vi "WPs and Obstacles 6.vi"(10 "WP Real Longs":dbl[](array[numeric])=[81.2671, 81.26711, 81.267112, 81.267332, 81.267916, 81.267137, 81.267874, 81.267301, 81.267913, 81.26772] format="%#_8g", 11 "WP Real Lats":dbl[](array[numeric])=[37.1528, 37.15281, 37.152877, 37.152903, 37.152565, 37.152792, 37.152806, 37.152779, 37.152868, 37.152484] format="%#_8g") -> (0 "Obstacle Real Lats and Longs":cluster{"Obs Lats":dbl[], "Obs Longs":dbl[]} {"Obs Longs" format="%#_8g"; "Obs Lats" format="%#_8g"}, 1 "WP Real Lats and Longs":cluster{"WP Lats":dbl[], "WP Longs":dbl[]} {"WP Longs" format="%#_8g"; "WP Lats" format="%#_8g"}, 2 "Sim Matrx":u8[][](array[numeric]), 3 "Real WP Map":T1(graph), 5 "Sim Course":picture)   [LabVIEW 2014]
panel:
  out "Array":dbl[](array[numeric])
  in  "Obstacle Real Longs":dbl[](array[numeric])=[81.2678, 81.267312, 81.267112, 81.267332, 81.267916, 81.267137, 81.267874, 81.267301, 81.267913, 81.26772] format="%#_8g"
  in  "Obstacle Real Lats":dbl[](array[numeric])=[37.1524, 37.152256, 37.152877, 37.152903, 37.152565, 37.152792, 37.152806, 37.152779, 37.152868, 37.152484] format="%#_8g"
  # "Waypoint and Obstacles 6 (Uses Paint and On-Screen WPs)"
  # "Added Global sim painted map"
  # "Inputs:"
  # "Sim Lats and Longs not being used"
  # "20"
  # "12"
  # "Outputs:"
  # "Sim Painted Picture to matrix"
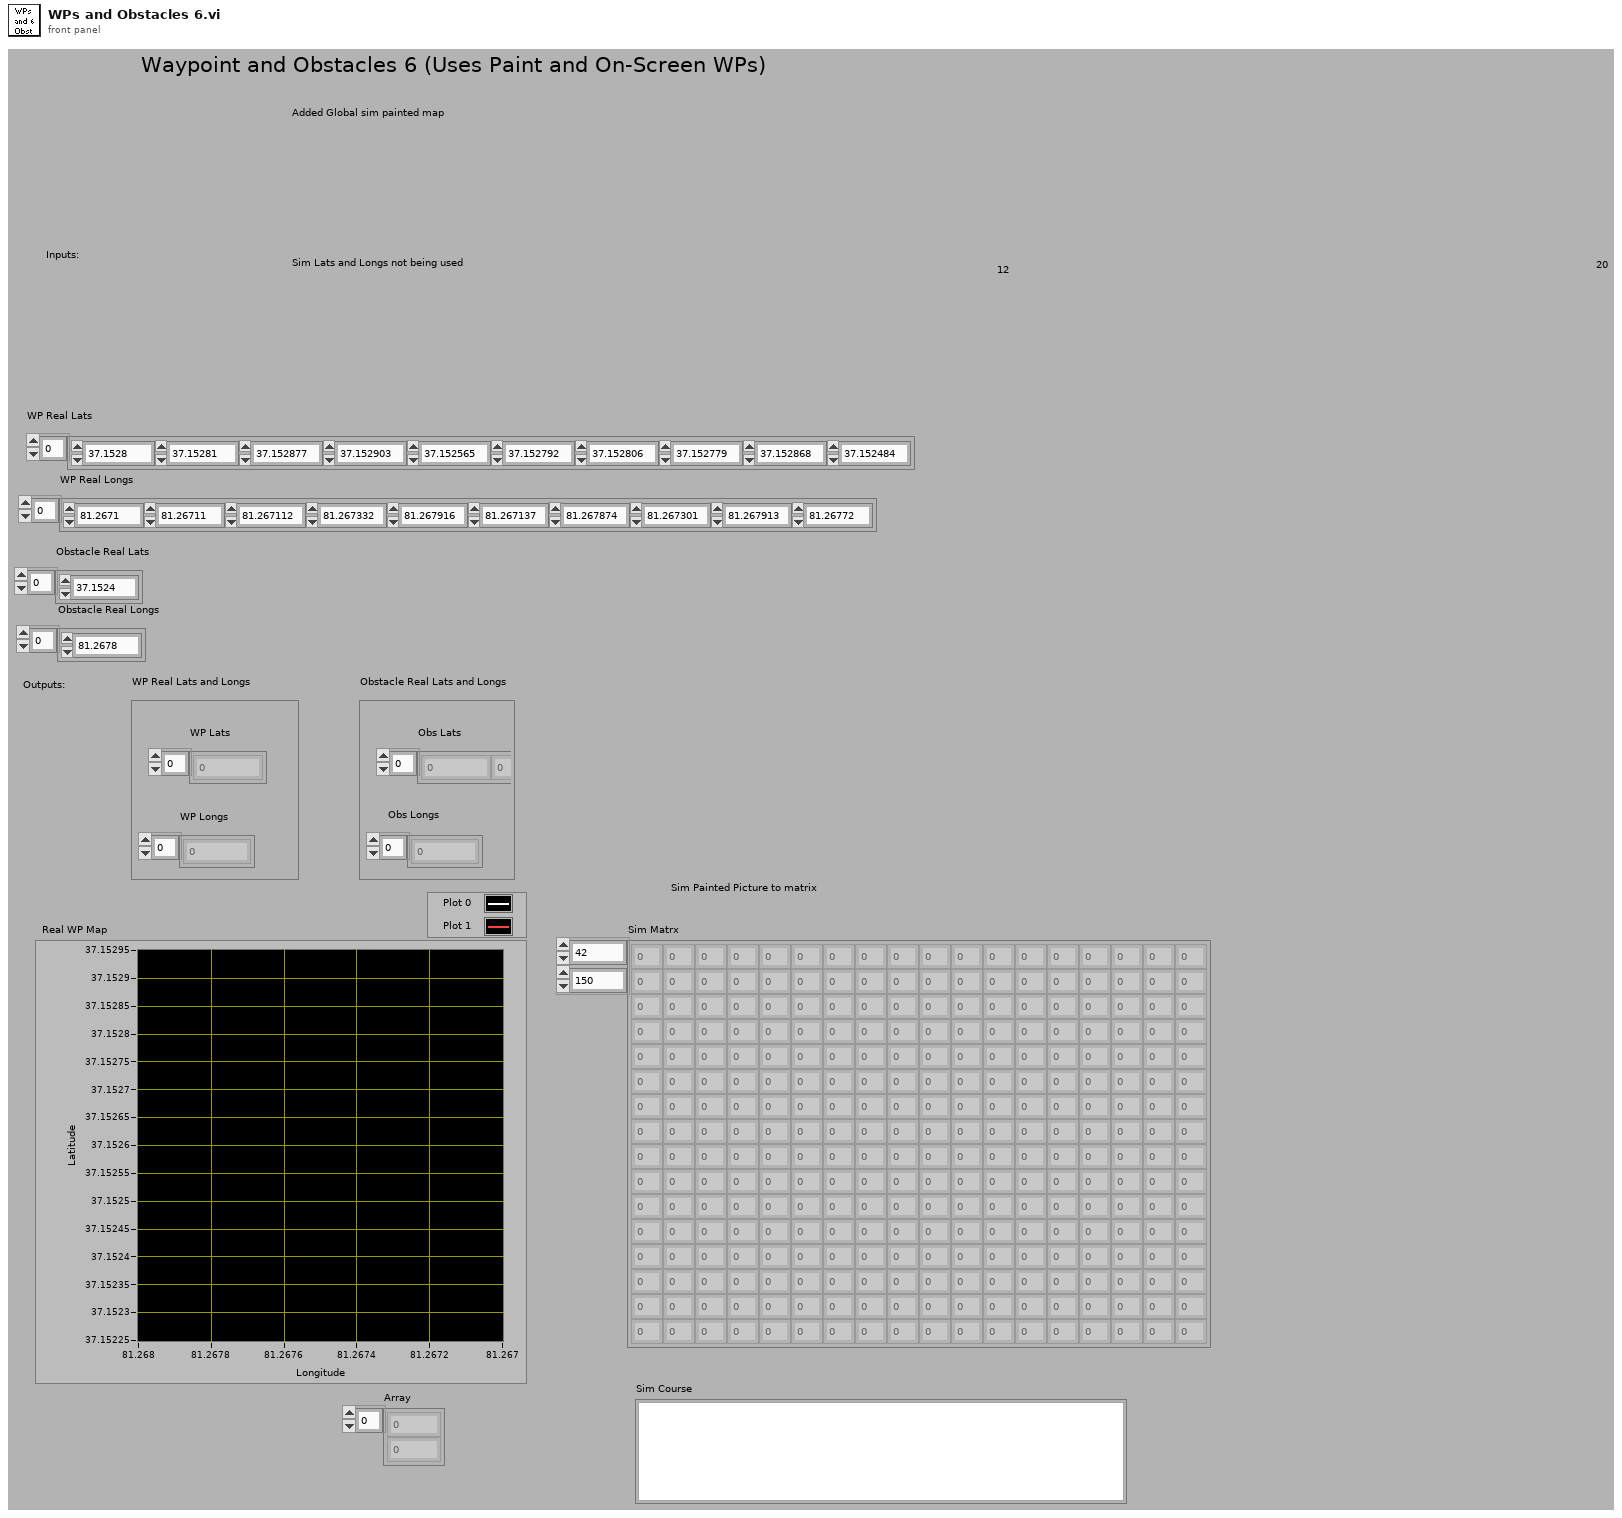
[diagram p1: front panel]
types:
  T1 = cluster{"Obstacle Longs":dbl[], "Obstacle Lats":dbl[]}[]
  T2 = cluster{"Obstacle Real Lats":dbl[], "Obstacle Real Longs":dbl[]}
  T3 = cluster{"WP Real Lats":dbl[], "WP Real Longs":dbl[]}
  T4 = cluster{"Obstacle Longs":dbl[], "Obstacle Lats":dbl[]}
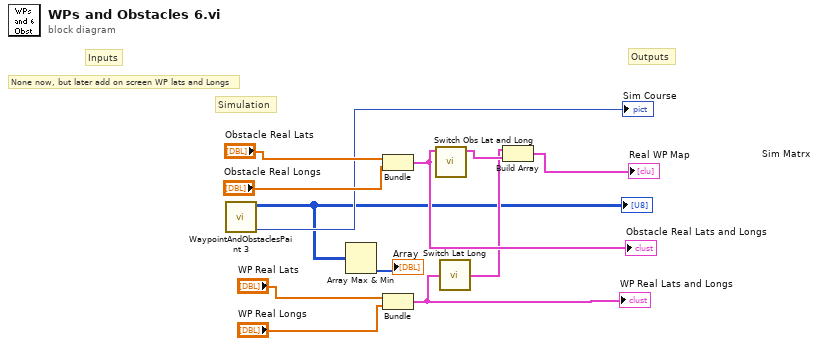
[diagram p0: block diagram]
diagram:
  # "None now, but later add on screen WP lats and Longs"
  # "Simulation"
  # "Inputs"
  # "Outputs"
  n1 = call "WaypointAndObstaclesPaint 3.vi"() -> ("Sim Course"=→"Sim Course":picture, 3:w2:u8[][])  [unwired: 10 in]
  "Sim Matrx" <- w2
  n2 = Array Max & Min(array=w2) -> (min index (indices)=→"Array":i32[])  [unwired: 3 out]
  n3 = Bundle("Obstacle Real Lats"="Obstacle Real Lats", "Obstacle Real Longs"="Obstacle Real Longs") -> (w11:T2)  [unwired: 1 in]
  "Obstacle Real Lats and Longs" <- w11
  n4 = Bundle("WP Real Lats"="WP Real Lats", "WP Real Longs"="WP Real Longs") -> (w12:T3)  [unwired: 1 in]
  "WP Real Lats and Longs" <- w12
  n5 = call "Switch Obs Lat and Long.vi"("Obstacle Lats and Longs for GIC"=w11) -> ("Obstacle Lats and Longs switched"=w10:T4)  [unwired: 10 in]
  n6 = call "Switch Lat Long.vi"("WP Lats and Longs for GIC"=w12) -> ("WP Lats and Longs switched"=w9:cluster{"WP Longs":dbl[], "WP Lats":dbl[]})
  n7 = Build Array(w9, w10) -> (→"Real WP Map":T1)
